vi "Write Shuffle Test Methods.vi"(8 "error in (no error)":errorcluster, 10 "Shuffle Test Methods":bool, 11 "Slave Test Runner In":refnum<class "Slave Test Runner.lvclass">) -> (0 "error out":errorcluster, 3 "Slave Test Runner Out":refnum<class "Slave Test Runner.lvclass">)   [LabVIEW 2020, in "Slave Test Runner.lvclass"]
uses:
  Slave Test Runner.lvclass
  Slave Test Runner.lvclass/Slave Test Runner.ctl
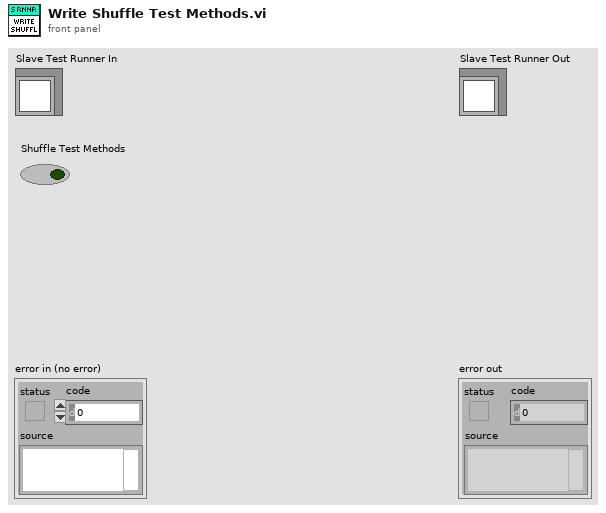
[diagram p1: front panel]
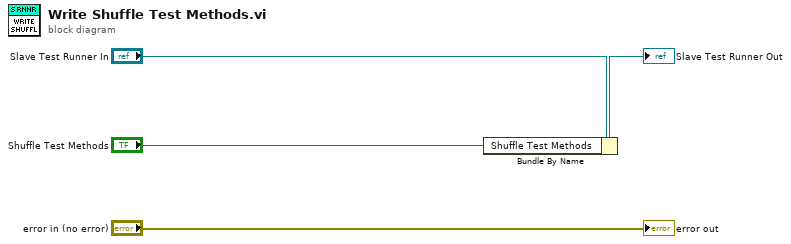
[diagram p0: block diagram]
diagram:
  n1 = Bundle By Name(cluster="Slave Test Runner In", "Shuffle Test Methods"="Shuffle Test Methods") -> (→"Slave Test Runner Out":refnum<class "Slave Test Runner.lvclass">)
  "error out" <- "error in (no error)"
